vi "visa read.vi"(8 "error in":errorcluster, 10 "delay before read (ms)":u32=500, 11 "VISA resource name in":refnum<visa-resource-name>) -> (0 "error out":errorcluster, 1 "return count":dbl, 2 "number":dbl format="%#.6f", 3 "VISA resource name out":refnum<visa-resource-name>)   [LabVIEW 2015, in "485 comm Custom Device.lvlib"]
doc: "This example performs a serial port write and a serial port read. The parameters set for the serial port must match the parameters of the connected instrument or device. The VISA Configure Serial Port VI sets the configuration parameters. The front panel displays the controls used to configure the basic parameters, such as baud rate, data bits, and parity. The VI passes the VISA resource name to other VIs that perform operations on that VISA resource. The VISA Write function sends a command to the serial device and the VISA Read function returns data based on the command. The VISA Close function then closes the reference to the serial device. It is important to close the reference; otherwise, further communication through that port might not be possible."
uses:
  485 comm Custom Device.lvlib
panel:
  out "bytes read":u32
  out "Response":string
  # "Overview: Demonstrates the use of the VISA functions to send a single command to a serial instrument and read a response.\nRequirements: NI-VISA Driver\nInstructions:\n1. Ensure the resource specified by the VISA resource name is a valid serial device.\n2. Run the VI.\n3. If your instrument recognizes the \"*IDN?\" command, it should return a Response."
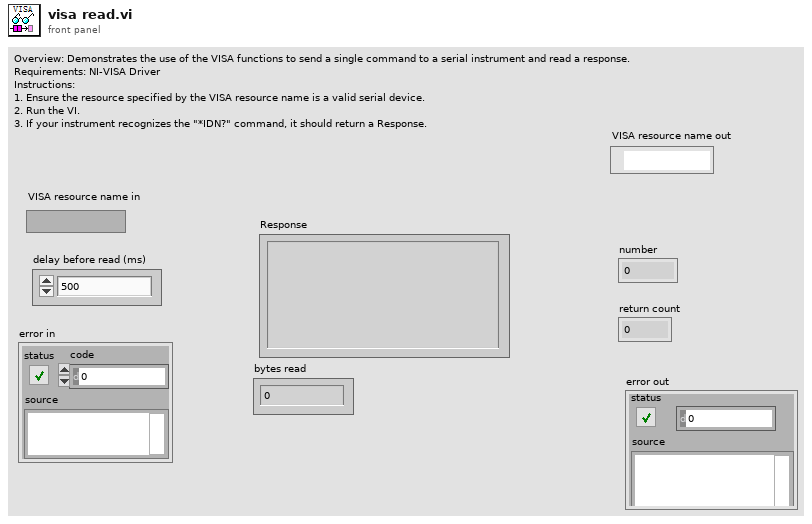
[diagram p1: front panel]
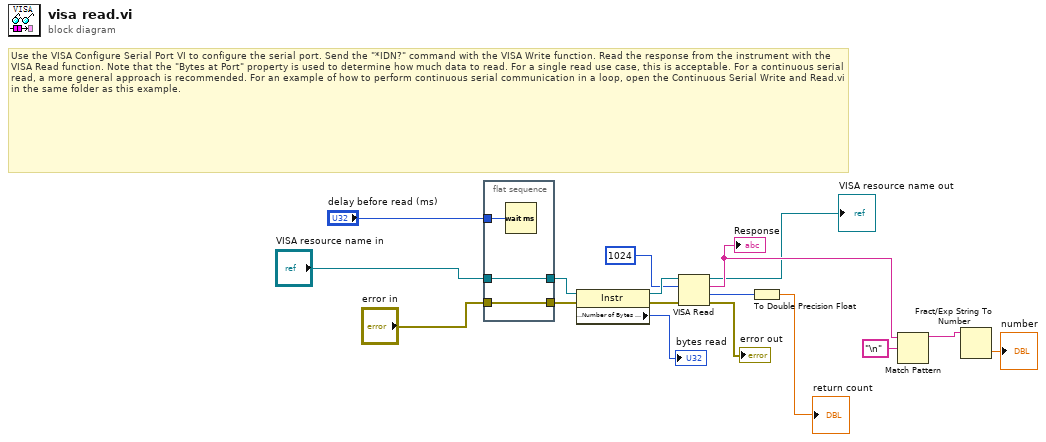
[diagram p0: block diagram]
diagram:
  # "Use the VISA Configure Serial Port VI to configure the serial port. Send the \"*IDN?\" command with the VISA Write function. Read the response from the instrument with the VISA Read function. Note that the \"Bytes at Port\" property is used to determine how much data to read. For a single read use case, this is acceptable. For a continuous serial read, a more general approach is recommended. For an example of how to perform continuous serial communication in a loop, open the Continuous Serial Write and Read.vi in the same folder as this example."
  n1 = flat-sequence {
    tunnel: "error in" -> [w19]
    tunnel: [w19] -> w17
    tunnel: "VISA resource name in" -> [w18]
    tunnel: [w18] -> w16
    tunnel: "delay before read (ms)" -> [w20]
    frame #0 {
      n2 = Wait (ms)(milliseconds to wait=w20) -> ()  [unwired: 1 out]
    }
  }
  n3 = property class="Instr"(reference=w16, error in=w17) -> (reference out=w14:refnum<visa-resource-name>, error out=w13:errorcluster, "Serial Settings:Number of Bytes at Serial Port"=→"bytes read":u32)
  n4 = VISA Read(VISA resource name=w14, byte count=u32 1024, error in (no error)=w13) -> (VISA resource name out=→"VISA resource name out":refnum<visa-resource-name>, read buffer=w8:string, return count=w6:u32, error out=→"error out":errorcluster)
  "Response" <- w8
  n5 = To Double Precision Float(number=w6) -> (double precision float=→"return count":dbl)
  n6 = Match Pattern(string=w8, regular expression="\n") -> (before substring=w9:string)  [unwired: 1 in, 3 out]
  n7 = Fract/Exp String To Number(string=w9) -> (number=→"number":dbl)  [unwired: 3 in, 1 out]
